vi "Multiplot-Disable.vi"() -> ()   [LabVIEW 2014]
panel:
  in  "stop":bool
  in  "Plot 2 disable":bool
  in  "Plot 1 disable":bool
  in  "Plot 0 disable":bool
  out "Waveform Graph":dynamicdata(graph)
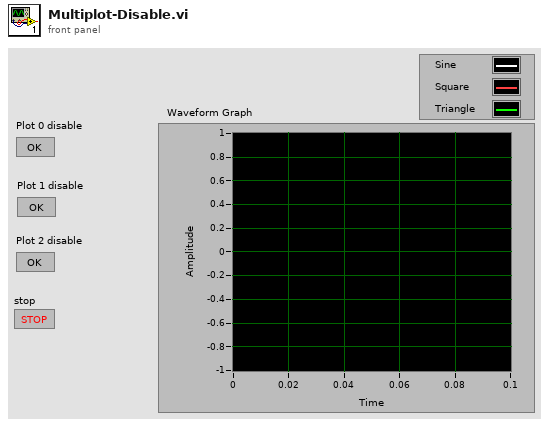
[diagram p1: front panel]
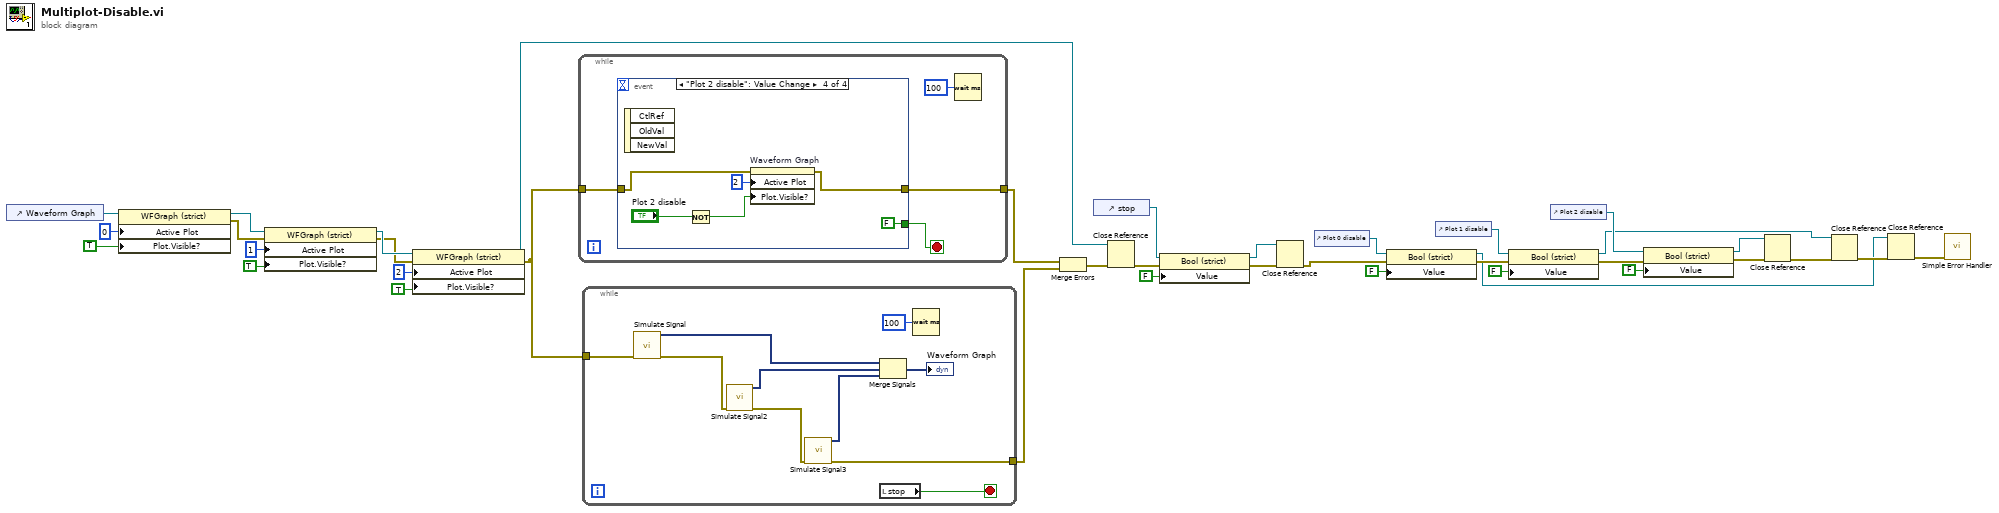
[diagram p0: block diagram]
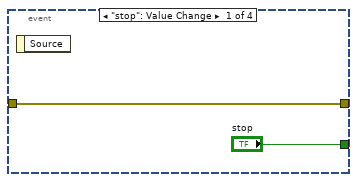
[diagram p2: hidden frame]
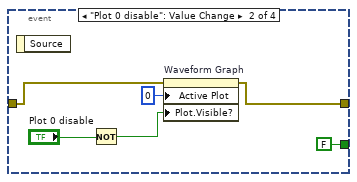
[diagram p3: hidden frame]
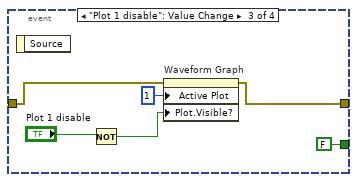
[diagram p4: hidden frame]
diagram:
  n1 = control-ref of="Waveform Graph"() -> (w37:refnum<vi>)
  n2 = property class="WFGraph (strict)"(reference=w37, "Active Plot"=u32 0, "Plot.Visible?"=TRUE ("Plot.Visible")) -> (reference out=w33:refnum<vi>, error out=w34:errorcluster)  [unwired: 1 in]
  n3 = property class="WFGraph (strict)"(reference=w33, error in=w34, "Active Plot"=u32 1, "Plot.Visible?"=TRUE ("Plot.Visible")) -> (reference out=w30:refnum<vi>, error out=w29:errorcluster)
  n4 = property class="WFGraph (strict)"(reference=w30, error in=w29, "Active Plot"=u32 2, "Plot.Visible?"=TRUE ("Plot.Visible")) -> (reference out=w22:refnum<vi>, error out=w26:errorcluster)
  n5 = while {
    tunnel: w26 -> [w40]
    tunnel: [w39] -> w24
    stop <- w41 stop-if-true
    n6 = event shown="[3] \"Plot 2 disable\": Value Change" {
      selector: _ -> [_ _ _ _]
      dyn-events: _ -> [_ _ _ _]
      timeout: _ -> [_ _ _ _]
      tunnel: ["stop" FALSE ("stop 3") FALSE ("stop 3") FALSE ("stop 3")] -> w41
      tunnel: w40 -> [w42 w49 w55 w61]
      tunnel: [w42 w48 w54 w60] -> w39
      event "stop": Value Change {
        n7 = event-data() -> ()  [unwired: 1 in, 1 out]
      }
      event "Plot 0 disable": Value Change {
        n8 = event-data() -> ()  [unwired: 1 in, 1 out]
        n9 = Not(x="Plot 0 disable") -> (.not. x?=w46:bool)
        n10 = property on="Waveform Graph" class="WFGraph (strict)"(error in=w49, "Active Plot"=u32 0, "Plot.Visible?"=w46) -> (error out=w48:errorcluster)  [unwired: 1 in, 1 out]
      }
      event "Plot 1 disable": Value Change {
        n11 = event-data() -> ()  [unwired: 1 in, 1 out]
        n12 = Not(x="Plot 1 disable") -> (.not. x?=w52:bool)
        n13 = property on="Waveform Graph" class="WFGraph (strict)"(error in=w55, "Active Plot"=u32 1, "Plot.Visible?"=w52) -> (error out=w54:errorcluster)  [unwired: 1 in, 1 out]
      }
      event "Plot 2 disable": Value Change {
        n14 = event-data() -> ()  [unwired: 1 in, 3 out]
        n15 = Not(x="Plot 2 disable") -> (.not. x?=w58:bool)
        n16 = property on="Waveform Graph" class="WFGraph (strict)"(error in=w61, "Active Plot"=u32 2, "Plot.Visible?"=w58) -> (error out=w60:errorcluster)  [unwired: 1 in, 1 out]
      }
    }
    n17 = Wait (ms)(milliseconds to wait=u32 100) -> ()  [unwired: 1 out]
  }
  n18 = while {
    tunnel: w26 -> [w71]
    tunnel: [w63] -> w25
    stop <- w65 stop-if-true
    n19 = call "Simulate Signal"("error in (no error)"=w71) -> ("Sine"=w68:dynamicdata, "error out"=w70:errorcluster)  [unwired: 13 in]
    n20 = call "Simulate Signal2"("error in (no error)"=w70) -> ("Square"=w67:dynamicdata, "error out"=w69:errorcluster)  [unwired: 13 in]
    n21 = call "Simulate Signal3"("error in (no error)"=w69) -> ("Triangle"=w66:dynamicdata, "error out"=w63:errorcluster)  [unwired: 13 in]
    n22 = Merge Signals(w68, w67, w66) -> (→"Waveform Graph":dynamicdata)
    n23 = local read "stop"() -> (w65:bool)
    n24 = Wait (ms)(milliseconds to wait=u32 100) -> ()  [unwired: 1 out]
  }
  n25 = Merge Errors(w24, w25) -> (w23:errorcluster)
  n26 = control-ref of="stop"() -> (w21:refnum<vi>)
  n27 = Close Reference(reference=w22, error in (no error)=w23) -> (error out=w20:errorcluster)
  n28 = property class="Bool (strict)"(reference=w21, error in=w20, "Value"=FALSE) -> (reference out=w17:refnum<vi>, error out=w18:errorcluster)
  n29 = Close Reference(reference=w17, error in (no error)=w18) -> (error out=w15:errorcluster)
  n30 = control-ref of="Plot 0 disable"() -> (w16:refnum<vi>)
  n31 = property class="Bool (strict)"(reference=w16, error in=w15, "Value"=FALSE) -> (reference out=w2:refnum<vi>, error out=w12:errorcluster)
  n32 = control-ref of="Plot 1 disable"() -> (w13:refnum<vi>)
  n33 = property class="Bool (strict)"(reference=w13, error in=w12, "Value"=FALSE) -> (reference out=w3:refnum<vi>, error out=w9:errorcluster)
  n34 = control-ref of="Plot 2 disable"() -> (w10:refnum<vi>)
  n35 = property class="Bool (strict)"(reference=w10, error in=w9, "Value"=FALSE) -> (reference out=w4:refnum<vi>, error out=w7:errorcluster)
  n36 = Close Reference(reference=w4, error in (no error)=w7) -> (error out=w6:errorcluster)
  n37 = Close Reference(reference=w3, error in (no error)=w6) -> (error out=w5:errorcluster)
  n38 = Close Reference(reference=w2, error in (no error)=w5) -> (error out=w1:errorcluster)
  n39 = call <vilib>:"Simple Error Handler.vi"("error in (no error)"=w1) -> ()  [unwired: 4 in, 5 out]
